vi "Load Settings from XML.vi"(11 "Settings In":T1={"Camera Configuration"={"Camera Index"=0}, "Logging Configuration"={"Log File Base Path"=path ""}, "XYZ Configuration"={"VISA resource name"="", "Timeout (3sec)"=0}, "DM Configuration"={"Selected Profile"="", "dm out"={"type"=0, "ID"=0, "size"=0, "@dummy control@"=0, "@dummy control@"=0, "@dummy control@"=0, "@dummy control@"=0, "lutName"=0}}, "Automation Configuration"={" Index"=0}, "V7001 Configuration"={" Index"=0}, "AOD Configuration"={"Physical Channel"="Dev1/ao0:1", "Maximum Value"=0.0, "Minimum Value"=1.0, "Update Rate"=192000.0}} {"AOD Configuration"."Update Rate" format="%0.2f"; "AOD Configuration"."Minimum Value" format="%0.2f"; "AOD Configuration"."Maximum Value" format="%0.2f"}) -> (3 "Settings Out":T1={"Camera Configuration"={"Camera Index"=0}, "Logging Configuration"={"Log File Base Path"=path ""}, "XYZ Configuration"={"VISA resource name"="", "Timeout (3sec)"=0}, "DM Configuration"={"Selected Profile"="", "dm out"={"type"=0, "ID"=0, "size"=0, "@dummy control@"=0, "@dummy control@"=0, "@dummy control@"=0, "@dummy control@"=0, "lutName"=0}}, "Automation Configuration"={" Index"=0}, "V7001 Configuration"={" Index"=0}, "AOD Configuration"={"Physical Channel"="Dev1/ao0:1", "Maximum Value"=0.0, "Minimum Value"=1.0, "Update Rate"=192000.0}} {"AOD Configuration"."Update Rate" format="%0.2f"; "AOD Configuration"."Minimum Value" format="%0.2f"; "AOD Configuration"."Maximum Value" format="%0.2f"})   [LabVIEW 2015, in "Settings.lvlib"]
uses:
  Settings.lvlib
  Settings.ctl
  Camera/Camera Configuration.ctl
  Logging/Logging Configuration.ctl
  XYZStage/XYZStage Configuration.ctl
  DM/DM Configuration.ctl
  Automation/Automation Configuration.ctl
  V7001/V7001 Configuration.ctl
  AOD/AOD Configuration.ctl
  <vilib>/Utility/xml.llb/Read From XML File(string).vi
  <vilib>/Utility/xml.llb/Write to XML File(string).vi
  Camera/Camera.lvlib
  Logging/Logging.lvlib
  XYZStage/XYZStage.lvlib
  DM/DM.lvlib
  Automation/Automation.lvlib
  V7001/V7001.lvlib
  AOD/AOD.lvlib
panel:
  in  "error in (no error)":errorcluster
  out "error out":errorcluster
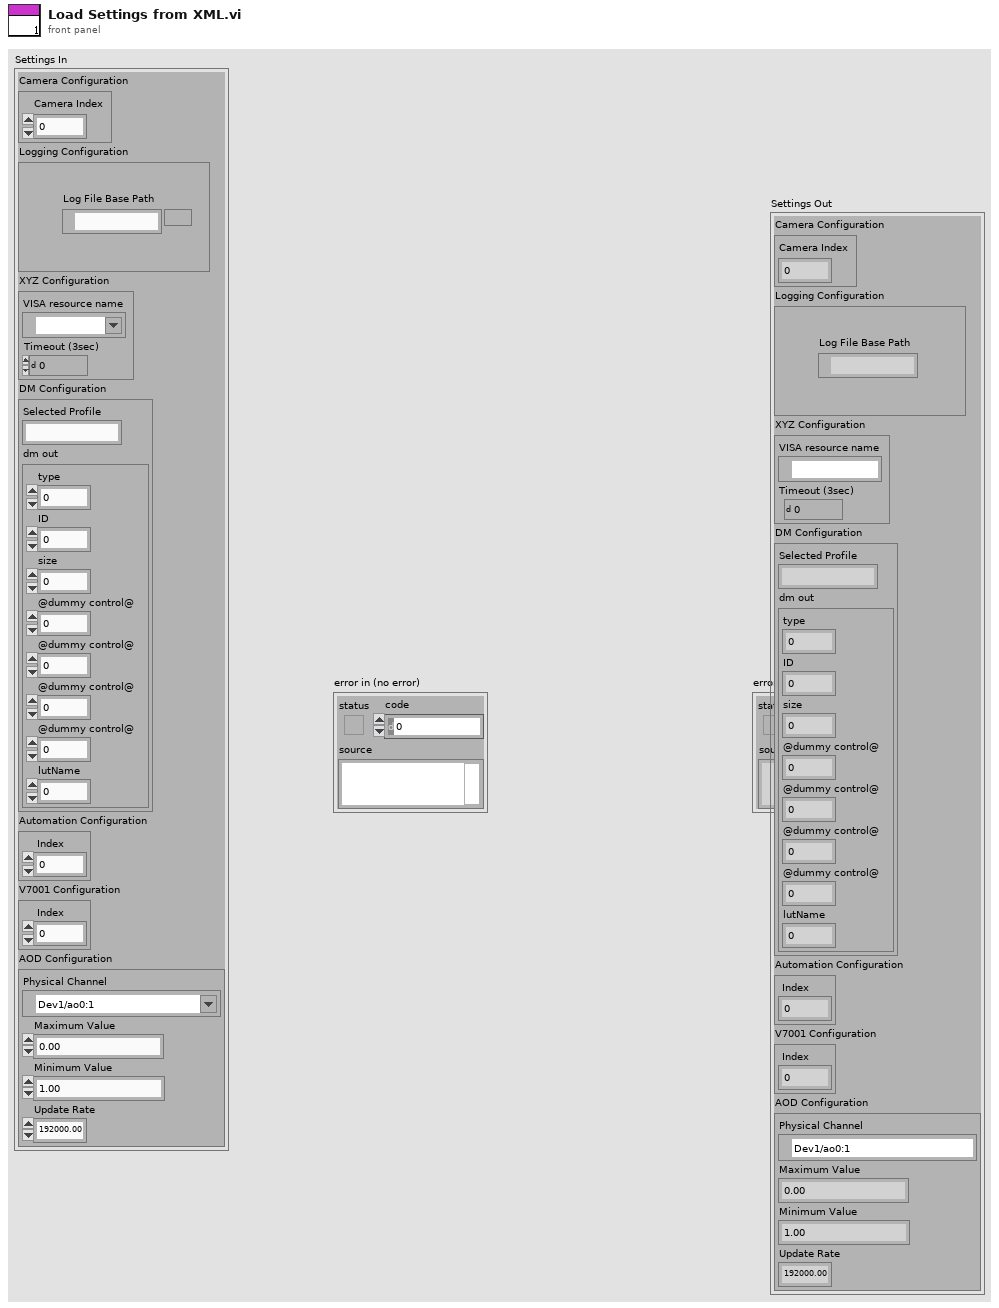
[diagram p1: front panel]
types:
  T1 = typedef "Settings.lvlib/Settings.ctl" = cluster{"Camera Configuration":T2, "Logging Configuration":T3, "XYZ Configuration":T4, "DM Configuration":T5, "Automation Configuration":T6, "V7001 Configuration":T7, "AOD Configuration":T8}
  T2 = typedef "Camera.lvlib/Camera Configuration.ctl" = cluster{"Camera Index":u32}
  T3 = typedef "Logging.lvlib/Logging Configuration.ctl" = cluster{"Log File Base Path":path}
  T4 = typedef "XYZStage.lvlib/XYZStage Configuration.ctl" = cluster{"VISA resource name":refnum<visa-resource-name>, "Timeout (3sec)":u32}
  T5 = typedef "DM.lvlib/DM Configuration.ctl" = cluster{"Selected Profile":string, "dm out":cluster{"type":i32, "ID":i32, "size":i32, "@dummy control@":i8, "@dummy control@":i8, "@dummy control@":i8, "@dummy control@":i8, "lutName":u64}}
  T6 = typedef "Automation.lvlib/Automation Configuration.ctl" = cluster{" Index":u32}
  T7 = typedef "V7001.lvlib/V7001 Configuration.ctl" = cluster{" Index":u32}
  T8 = typedef "AOD.lvlib/AOD Configuration.ctl" = cluster{"Physical Channel":tag, "Maximum Value":dbl, "Minimum Value":dbl, "Update Rate":dbl}
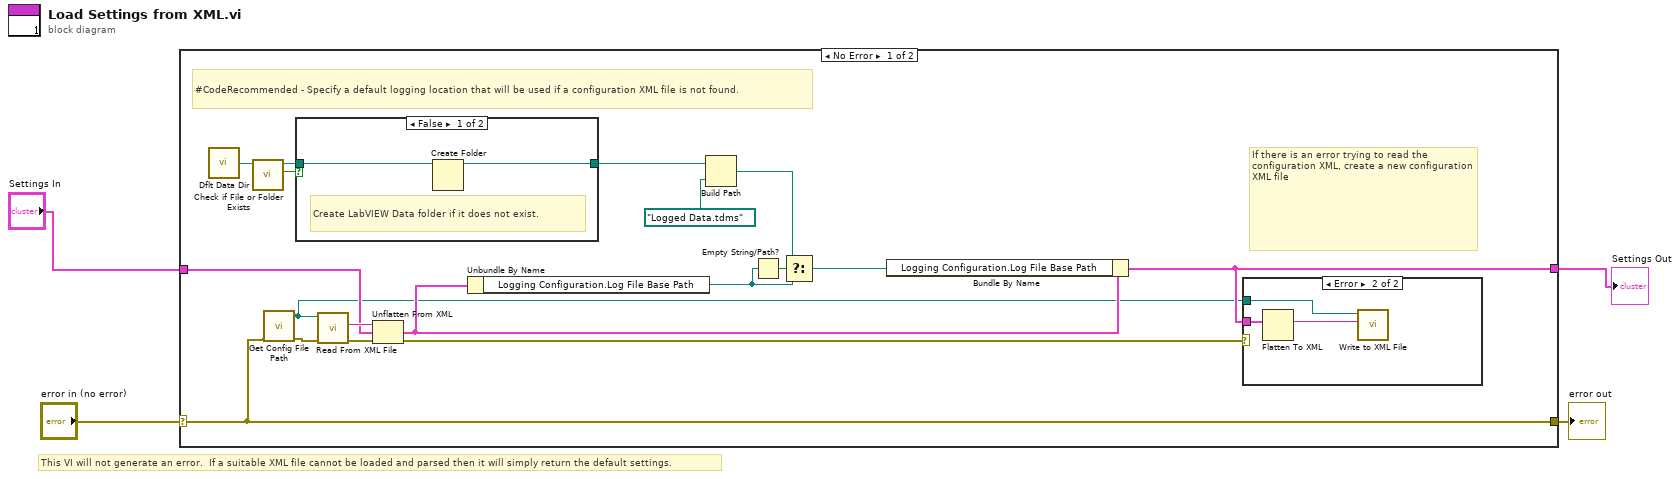
[diagram p0: block diagram]
diagram:
  # "This VI will not generate an error.  If a suitable XML file cannot be loaded and parsed then it will simply return the default settings."
  n1 = case shown="No Error" "error in (no error)" {
    selector: "error in (no error)" -> [w6 w30]
    tunnel: [w6 w30] -> w3
    tunnel: "Settings In" -> [w18 w29]
    tunnel: [w12 w29] -> w1
    frame No Error {
      # "If there is an error trying to read the configuration XML, create a new configuration XML file"
      # "#CodeRecommended - Specify a default logging location that will be used if a configuration XML file is not found."
      n2 = call <vilib>:"Dflt Data Dir.vi"() -> ("App:Default Data Directory"=w11:path)
      n3 = call <vilib>:"Check if File or Folder Exists.vi"("path"=w11) -> ("file or folder exists?"=w10:bool, "dup path"=w9:path)  [unwired: 8 in, 1 out]
      n4 = call "Get Config File Path.vi"("error in (no error)"=w6) -> ("error out"=w7:errorcluster, "XML File Path"=w5:path)  [unwired: 9 in]
      n5 = case shown="False" w10 {
        tunnel: w9 -> [w24 w25]
        tunnel: [w23 w25] -> w8
        frame False {
          # "Create LabVIEW Data folder if it does not exist."
          n6 = Create Folder(path (use dialog)=w24) -> (created path=w23:path)  [unwired: 2 in, 2 out]
        }
        frame True {
        }
      }
      n7 = call-poly <vilib>:"Read From XML File.vi"("error in (no error)"=w7, "XML File Path"=w5) -> ("error out"=w20:errorcluster, "XML Elements"=w22:string)  [unwired: 7 in, 1 out]
      n8 = Unflatten From XML(xml string=w22, type=w18, error in (no error)=w20) -> (value=w14:T1, error out=w19:errorcluster)
      n9 = Unbundle By Name(w14) -> ("Logging Configuration.Log File Base Path"=w16:path)
      n10 = Build Path(base path=w8, name or relative path=path "Logged Data.tdms" ("App:Default Data Directory")) -> (appended path=w15:path)
      n11 = Empty String/Path?(string/path=w16) -> (empty?=w17:bool)
      n12 = Select(t=w15, s=w17, f=w16) -> (s? t:f=w13:path)
      n13 = Bundle By Name(cluster=w14, "Logging Configuration.Log File Base Path"=w13) -> (w12:T1)
      n14 = case shown="Error" w19 {
        tunnel: w12 -> [_ w28]
        tunnel: w5 -> [_ w26]
        frame No Error {
        }
        frame Error {
          n15 = Flatten To XML(anything=w28) -> (xml string=w27:string)
          n16 = call-poly <vilib>:"Write to XML File.vi"("XML Input"=w27, "XML File Path"=w26) -> ()  [unwired: 7 in, 3 out]
        }
      }
    }
    frame Error {
    }
  }
  "error out" <- w3
  "Settings Out" <- w1
